vi "Light-emitting Diode.vi"(8 "error in":errorcluster) -> (0 "error out":errorcluster, 2 "Pass?":bool, 3 "VISA resource name out":refnum<visa-resource-name>, 5 "R Pass/fai":bool, 7 "G Pass/fail":bool)   [LabVIEW 2009]
uses:
  Digit IO PCI 6503/Digit IO control.ctl
  Global/Global 1.vi
  <vilib>/Instr/_visa.llb/VISA Configure Serial Port (Instr).vi
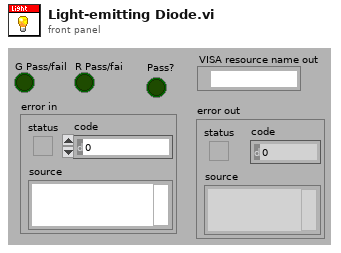
[diagram p1: front panel]
types:
  T1 = typedef "Digit IO control.ctl" = enum16{"Pull X1_4 Low", "Disconnect Pull X1_4 Low", "Down Cylinder", "Disconnect Down Cylinder", "Load X1_1_5", "Disconnect Load X1_1_5", "Measu X1_1_5", "Disconnect Measu X1_1_5", "Measu Z1_1_5", "Disconnect Measu Z1_1_5", "Power X1_1", "Disconnect Power X1_1", "RS232 Power", "Disconnect RS232 Power", "Card Cylinder", "Disconnect Card Cylinder", "Fail LED", "Disconnect Fail LED", "LCA Power", "Disconnect LCA Power", "BeyondCylinderDowndigit", "Disconnect BeyondCylinderDowendigit", "Frequency", "Disconnect Frequency", "Measu Current", "Disconnect Measu Current", "Measu current_1", "Disconnect Measu current_1", "Digit ALL", "Disconnect Digit ALL", "PASS LED", "Disconnect PASS LED", "Load Z1_1_3", "Disconnect Load Z1_1_3", "RS232 Connect", "Disconnect RS232 Connect", "Power Z1_7", "Disconnect Power Z1_7", "Pull Z_1_5  low", "Disconnect Pull Z_1_5  low", "Connect LCA_1", "Disconnect LCA_1", "short LCA", "Disconnect short LCA", "PT100", "Disconnect PT100", "NO connect", "Disconnect NO connect"}
  T2 = enum16{"LCU Power on", "Command _G", "Verify Green light", "Command _g", "Green light Off", "Command _R", "Verify Red light", "Command _r", "Red light Off", "Finish"}
  T3 = cluster{"People":string, "product  number":string, "Test time":string, "VHeatFuse_noload":string, "VHeatFuse_load":string, "VoverrideDiode":string, "Test firmware upload via X1":string, "TemperAddress":string, "Troom":string, "TLCU":string, "Adjustment factor":string, "MeasuredFreq":string, "I2C communication":string, "Light-emitting diode on Z2":string, "Battery warning/inhibit":string, "Reset by IC10":string, "External EEPROM":string, "RFID card detection and reading RFID":string, "Production parameters in internal EEPROM":string, "Current consumption in sleep mode":string, "Application and database upload":string, "Test result":string, "Table head[22]":string, "Table head[23]":string}
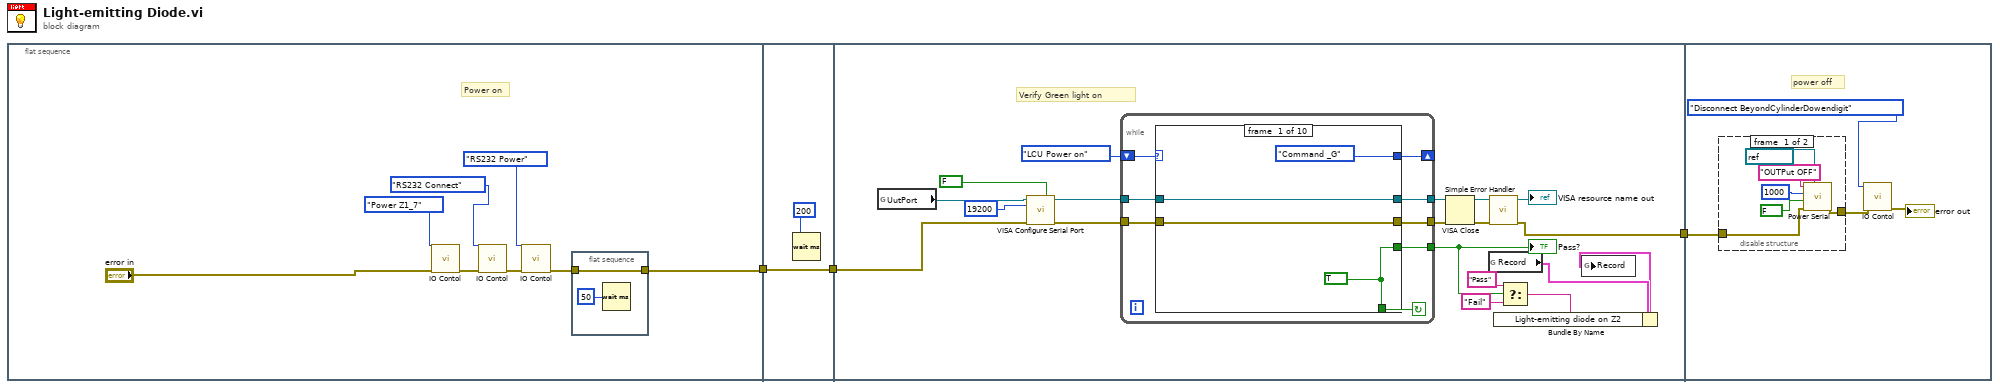
[diagram p0: block diagram]
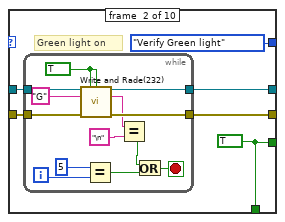
[diagram p2: hidden frame]
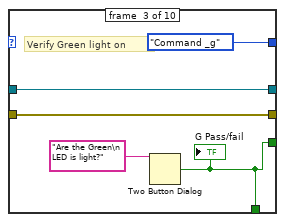
[diagram p3: hidden frame]
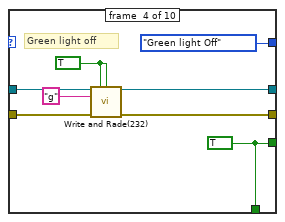
[diagram p4: hidden frame]
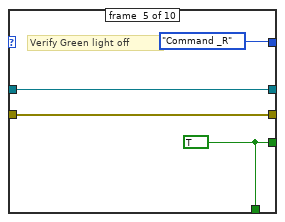
[diagram p5: hidden frame]
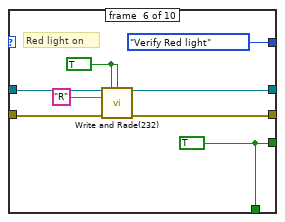
[diagram p6: hidden frame]
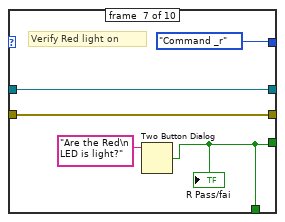
[diagram p7: hidden frame]
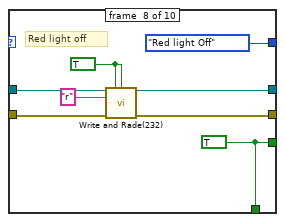
[diagram p8: hidden frame]
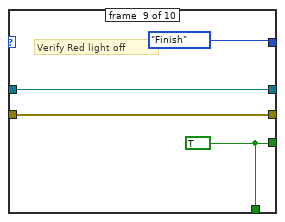
[diagram p9: hidden frame]
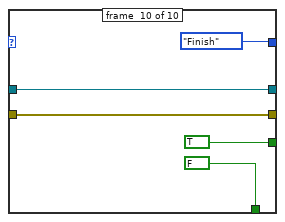
[diagram p10: hidden frame]
diagram:
  n1 = flat-sequence {
    tunnel: [w5] -> w1
    tunnel: [w14] -> w2
    tunnel: w1 -> [w14]
    tunnel: [w25] -> w3
    tunnel: w2 -> [w17]
    tunnel: w3 -> [w113]
    frame #0 {
      # "Power on"
      n2 = call "IO Contol.vi"("error in"="error in", "IO Operation"=Digit_IO_control."Power Z1_7" ("Enum")) -> ("error out"=w10:errorcluster)  [unwired: 9 out]
      n3 = call "IO Contol.vi"("error in"=w10, "IO Operation"=Digit_IO_control."RS232 Connect" ("Enum")) -> ("error out"=w11:errorcluster)  [unwired: 9 out]
      n4 = call "IO Contol.vi"("error in"=w11, "IO Operation"=Digit_IO_control."RS232 Power" ("Enum")) -> ("error out"=w6:errorcluster)  [unwired: 9 out]
      n5 = flat-sequence {
        tunnel: [w13] -> w5
        tunnel: w6 -> [w13]
        frame #0 {
          n6 = Wait (ms)(milliseconds to wait=u32 50) -> ()  [unwired: 1 out]
        }
      }
    }
    frame #1 {
      n7 = Wait (ms)(milliseconds to wait=u32 200) -> ()  [unwired: 1 out]
    }
    frame #2 {
      # "Verify Green light on"
      n8 = global read "Global 1.vi" "UutPort"() -> (w16:refnum<visa-resource-name>)
      n9 = call-poly "VISA Configure Serial Port"("VISA resource name"=w16, "Enable Termination\nChar (T)"=FALSE ("Enable Termination\nChar (T)"), "baud rate (9600)"=u32 19200, "error in (no error)"=w17) -> ("VISA resource name out"=w27:refnum<visa-resource-name>, "error out"=w24:errorcluster)  [unwired: 3 in, 7 out]
      n10 = while {
        shift-right: [w33] -> _
        shift-left: T2."LCU Power on" -> [w34]
        tunnel: [w39] -> w28
        tunnel: w27 -> [w38]
        tunnel: [w37] -> w26
        tunnel: w24 -> [w36]
        tunnel: [w35] -> w23
        stop <- w40 continue-if-true
        n11 = case shown="\"Verify Red light\"" w34 {
          tunnel: [T2."Command _G" T2."Verify Green light" T2."Command _g" T2."Green light Off" T2."Command _R" T2."Verify Red light" T2."Command _r" T2."Red light Off" T2."Finish" T2."Finish"] -> w33
          tunnel: [w42 w45 w64 w70 w77 w82 w89 w95 w102 FALSE] -> w40
          tunnel: [w44 w47 w68 w72 w80 w84 w93 w97 w104 w110] -> w39
          tunnel: w38 -> [w44 w50 w68 w74 w80 w86 w93 w99 w104 w110]
          tunnel: [w43 w48 w67 w71 w79 w83 w92 w96 w103 w109] -> w37
          tunnel: w36 -> [w43 w49 w67 w73 w79 w85 w92 w98 w103 w109]
          tunnel: [w42 w45 w64 w70 w77 w82 w89 w95 w102 TRUE] -> w35
          frame #0 {
            w42 = TRUE
          }
          frame #1 {
            w45 = TRUE ("write")
            # "Green light on"
            n12 = while {
              tunnel: w50 -> [w63]
              tunnel: w49 -> [w62]
              tunnel: [w59] -> w48
              tunnel: [w58] -> w47
              i -> [w54]
              stop <- w53 stop-if-true
              w61 = TRUE ("write")
              n13 = call "Write and Rade(232).vi"("VISA resource name in"=w63, "write"=w61, "read"=w61, "string to write"="G", "error in"=w62) -> ("VISA resource name out"=w58:refnum<visa-resource-name>, "read string"=w56:string, "error out"=w59:errorcluster)  [unwired: 3 in, 5 out]
              n14 = Equal?(x=5, y=w54) -> (x = y?=w51:bool)
              n15 = Equal?(x=w56, y="\n" ("string to write")) -> (x = y?=w52:bool)
              n16 = Or(x=w52, y=w51) -> (x .or. y?=w53:bool)
            }
          }
          frame #2 {
            # "Verify Green light on"
            n17 = Two Button Dialog(message="Are the Green\n LED is light?") -> (T button?=w64:bool)  [unwired: 2 out]
            "G Pass/fail" <- w64
          }
          frame #3 {
            w70 = TRUE ("write")
            w76 = TRUE ("write")
            # "Green light off"
            n18 = call "Write and Rade(232).vi"("VISA resource name in"=w74, "write"=w76, "read"=w76, "string to write"="g", "error in"=w73) -> ("VISA resource name out"=w72:refnum<visa-resource-name>, "error out"=w71:errorcluster)  [unwired: 3 in, 6 out]
          }
          frame #4 {
            w77 = TRUE
            # "Verify Green light off"
          }
          frame #5 {
            w82 = TRUE ("write")
            w88 = TRUE ("write")
            # "Red light on"
            n19 = call "Write and Rade(232).vi"("VISA resource name in"=w86, "write"=w88, "read"=w88, "string to write"="R", "error in"=w85) -> ("VISA resource name out"=w84:refnum<visa-resource-name>, "error out"=w83:errorcluster)  [unwired: 3 in, 6 out]
          }
          frame #6 {
            # "Verify Red light on"
            n20 = Two Button Dialog(message="Are the Red\n LED is light?") -> (T button?=w89:bool)  [unwired: 2 out]
            "R Pass/fai" <- w89
          }
          frame #7 {
            w95 = TRUE
            w101 = TRUE ("write")
            # "Red light off"
            n21 = call "Write and Rade(232).vi"("VISA resource name in"=w99, "write"=w101, "read"=w101, "string to write"="r", "error in"=w98) -> ("VISA resource name out"=w97:refnum<visa-resource-name>, "error out"=w96:errorcluster)  [unwired: 3 in, 6 out]
          }
          frame #8 {
            w102 = TRUE
            # "Verify Red light off"
          }
          frame #9 {
          }
        }
      }
      "VISA resource name out" <- w28
      "Pass?" <- w23
      n22 = VISA Close(VISA resource name=w28, error in (no error)=w26) -> (error out=w30:errorcluster)
      n23 = global read "Global 1.vi" "Record"() -> (w20:T3)
      n24 = call <vilib>:"Simple Error Handler.vi"("error in (no error)"=w30) -> ("error out"=w25:errorcluster)  [unwired: 1 in, 7 out]
      n25 = Select(t="Pass", s=w23, f="Fail") -> (s? t:f=w18:string)
      n26 = Bundle By Name(cluster=w20, "Light-emitting diode on Z2"=w18) -> (w19:T3)
      n27 = global write "Global 1.vi" "Record"(w19) -> ()
    }
    frame #3 {
      # "power off"
      n28 = disable-structure shown="Enabled" {
        disable-tunnel: w113 -> [w117 w121]
        disable-tunnel: [w116 w121] -> w112
        frame #0 {
          n29 = call "Power Serial.vi"("VISA Resource Address"=refnum<visa-resource-name> "COM1", "error in (no error)"=w117, "Rd?"=FALSE, "Delay"=1000, "IN"="OUTPut OFF" ("In")) -> ("error out"=w116:errorcluster)  [unwired: 5 in, 1 out]
        }
        frame #1 {
        }
      }
      n30 = call "IO Contol.vi"("error in"=w112, "IO Operation"=Digit_IO_control."Disconnect BeyondCylinderDowendigit" ("Enum")) -> ("error out"=→"error out":errorcluster)  [unwired: 9 out]
    }
  }
